vi "Locate P2.vi"(0 "Image In":T1, 11 "Error In":errorcluster, 13 "Template File Path (Locate P2 Hole)":path=path "C:/Users/serce/Desktop/Smart Vision System Testbench/P2/P2 Hole Template.png") -> (2 "Number of Matches (Locate P2 Hole)":i32, 4 "Image Dup Out":T1, 15 "Error Out":errorcluster)   [LabVIEW 2020, in "BilGör.lvlib"]
uses:
  <vilib>/vision/Image Controls.llb/IMAQ Image.ctl
  <vilib>/vision/Pattern Matching.llb/IMAQ Curve Parameters.ctl
  <vilib>/vision/Pattern Matching.llb/IMAQ Match Range Setting.ctl
  <vilib>/vision/Pattern Matching.llb/IMAQ Geometric Pattern 2 Advanced Match Options.ctl
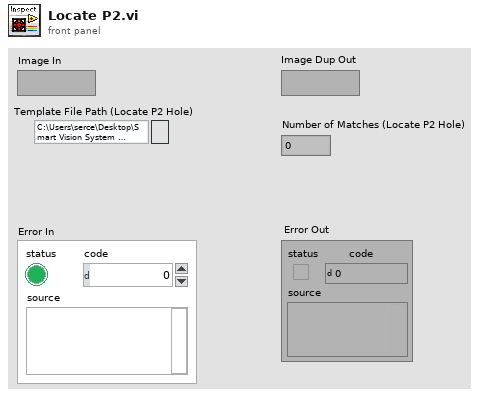
[diagram p1: front panel]
types:
  T1 = typedef "IMAQ Image.ctl" = refnum<image>
  T2 = typedef "IMAQ Curve Parameters.ctl" = cluster{"Extraction Mode":u32, "Edge Threshold":i32, "Edge Filter Size":u32, "Min Length":i32, "Row Search Step Size":i32, "Col Search Step Size":i32, "Max Endpoint Gap":i32, "Closed":bool, "Subpixel":bool}
  T3 = typedef "IMAQ Match Range Setting.ctl" = cluster{"Match Constraints":u32, "Min":dbl, "Max":dbl}
  T4 = typedef "IMAQ Geometric Pattern 2 Advanced Match Options.ctl" = u16
  T5 = cluster{"Curve Parameters":T2, "Match Mode":cluster{"Rotation":bool, "Scale":bool, "Occlusion":bool, "Reserved 1":bool, "Reserved 2":bool, "Reserved 3":bool}, "Range Settings":T3[], "Number of Matches":i32, "Minimum Match Score":sgl, "SubPixel Accuracy":bool, "Adv. Geometric Match Options 2":cluster{"Setup Data Item":T4, "Item Value":dbl}[]}
  T6 = enum16{"Reset", "Update Coordinate System", "Get Coordinate System"}
  T7 = enum16{"Horizontal Motion", "Vertical Motion", "Horizontal and Vertical Motion", "Horizontal, Vertical and Angular Motion"}
  T8 = cluster{"Origin":cluster{"X":sgl, "Y":sgl}, "Angle (deg)":sgl, "Axis Reference":u32}
  T9 = cluster{"Global Rectangle":i32[], "Contours":cluster{"ID":enum32{"External", "Internal"}, "Type":u32, "Coordinates":i32[]}[]}
  T10 = typedef "IMAQ GM Match Report.ctl" = cluster{"Position":cluster{"x":sgl, "y":sgl}, "Angle":sgl, "Scale":sgl, "Score":sgl, "Bounding Box":cluster{"x":sgl, "y":sgl}[], "Contrast Reversed":bool, "Occlusion %":sgl, "Template Target Curve Score":sgl, "Target Template Curve Score":sgl, "Correlation Score":sgl}
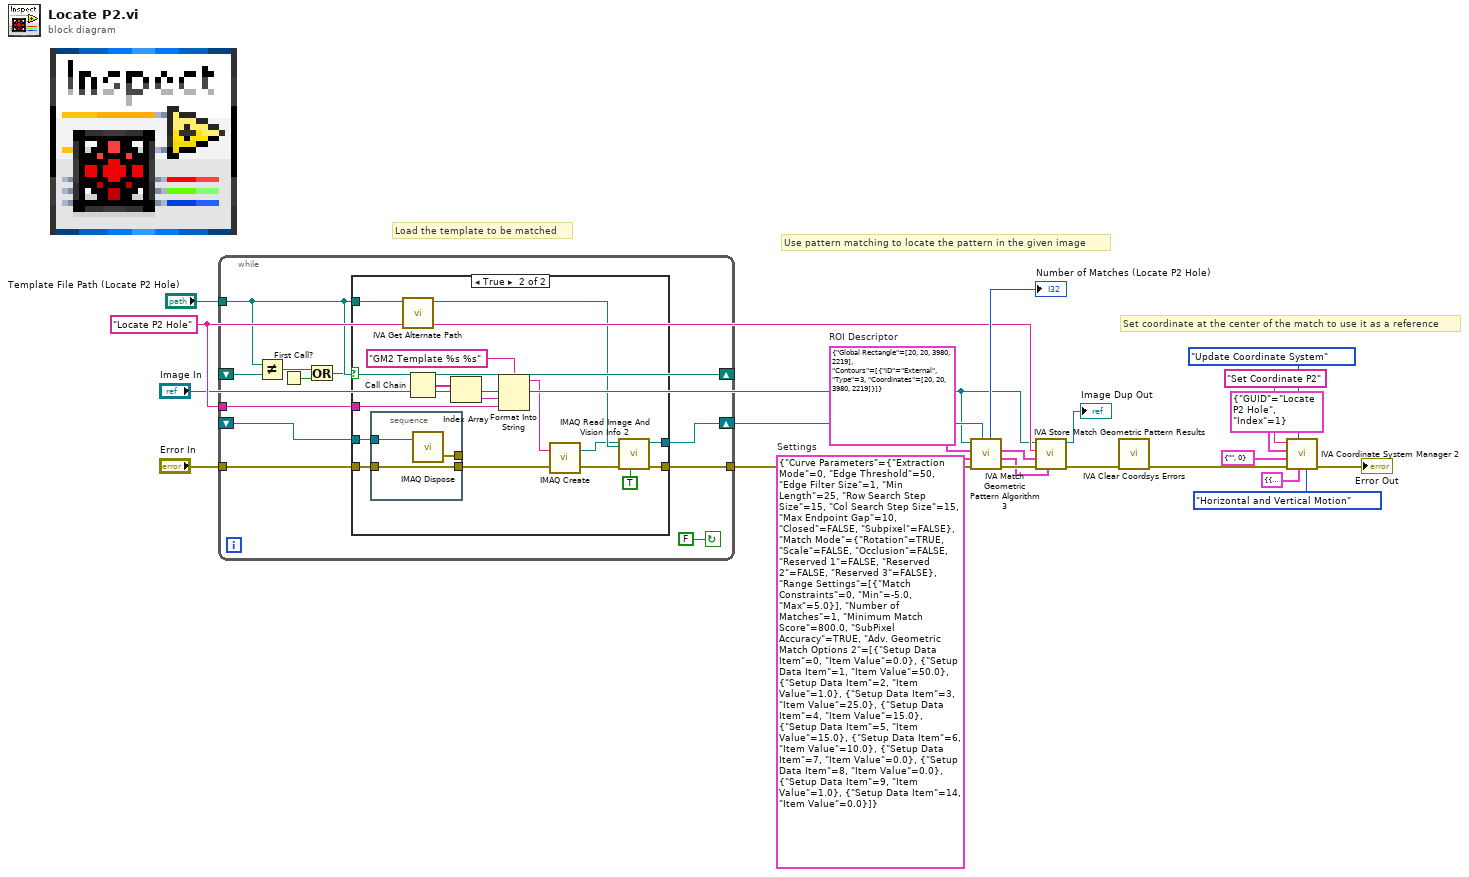
[diagram p0: block diagram]
diagram:
  w16 = T5 {"Curve Parameters"={"Extraction Mode"=0, "Edge Threshold"=50, "Edge Filter Size"=1, "Min Length"=25, "Row Search Step Size"=15, "Col Search Step Size"=15, "Max Endpoint Gap"=10, "Closed"=FALSE, "Subpixel"=FALSE}, "Match Mode"={"Rotation"=TRUE, "Scale"=FALSE, "Occlusion"=FALSE, "Reserved 1"=FALSE, "Reserved 2"=FALSE, "Reserved 3"=FALSE}, "Range Settings"=[{"Match Constraints"=0, "Min"=-5.0, "Max"=5.0}], "Number of Matches"=1, "Minimum Match Score"=800.0, "SubPixel Accuracy"=TRUE, "Adv. Geometric Match Options 2"=[{"Setup Data Item"=0, "Item Value"=0.0}, {"Setup Data Item"=1, "Item Value"=50.0}, {"Setup Data Item"=2, "Item Value"=1.0}, {"Setup Data Item"=3, "Item Value"=25.0}, {"Setup Data Item"=4, "Item Value"=15.0}, {"Setup Data Item"=5, "Item Value"=15.0}, {"Setup Data Item"=6, "Item Value"=10.0}, {"Setup Data Item"=7, "Item Value"=0.0}, {"Setup Data Item"=8, "Item Value"=0.0}, {"Setup Data Item"=9, "Item Value"=1.0}, {"Setup Data Item"=14, "Item Value"=0.0}]}  # Settings
  w15 = "Locate P2 Hole" ("Step Name")
  w21 = T9 {"Global Rectangle"=[20, 20, 3980, 2219], "Contours"=[{"ID"=enum."External", "Type"=3, "Coordinates"=[20, 20, 3980, 2219]}]}  # ROI Descriptor
  # "Set coordinate at the center of the match to use it as a reference"
  # "Use pattern matching to locate the pattern in the given image"
  # "Load the template to be matched"
  n1 = while {
    shift-right: [w33] -> w13
    shift-left: _ -> [w32]
    tunnel: [w30] -> w14
    tunnel: "Error In" -> [w29]
    tunnel: "Template File Path (Locate P2 Hole)" -> [w26]
    tunnel: w15 -> [w28]
    shift-right: [w26] -> _
    shift-left: _ -> [w27]
    stop <- FALSE continue-if-true
    n2 = Not Equal?(x=w26, y=w27) -> (x != y?=w24:bool)
    n3 = First Call?() -> (First Call?: T/F=w25:bool)
    n4 = Or(x=w24, y=w25) -> (x .or. y?=w23:bool)
    n5 = case shown="True" w23 {
      tunnel: [w35 w37] -> w33
      tunnel: w32 -> [w35 w44]
      tunnel: [w34 w39] -> w30
      tunnel: w29 -> [w34 w45]
      tunnel: w28 -> [_ w46]
      tunnel: w26 -> [_ w43]
      frame False {
      }
      frame True {
        n6 = stacked-sequence {
          tunnel: w45 -> [w53]
          tunnel: w44 -> [w52]
          tunnel: [w53] -> w42
          tunnel: [w51] -> _
          frame #0 {
            n7 = call "IMAQ Dispose"("Image"=w52) -> ("error out"=w51:errorcluster)  [unwired: 2 in, 3 out]
          }
        }
        n8 = call <vilib>:"IVA Get Alternate Path.vi"("Path In"=w43) -> ("Path Out"=w38:path)  [unwired: 10 out]
        n9 = Call Chain() -> (call chain=w48:string[])
        n10 = Index Array(array=w48) -> (element=w47:string)  [unwired: 1 in]
        n11 = Format Into String(format string="GM2 Template %s %s" ("Image Name"), w47, w46) -> (resulting string=w50:string)  [unwired: 2 in, 1 out]
        n12 = call "IMAQ Create"("Image Name"=w50, "error in (no error)"=w42) -> ("New Image"=w36:T1, "error out"=w40:errorcluster)  [unwired: 2 in, 1 out]
        n13 = call "IMAQ Read Image And Vision Info 2"("Use File Path Image Type"=TRUE, "File Path"=w38, "error in (no error)"=w40, "Image"=w36) -> ("error out"=w39:errorcluster, "Image Out"=w37:T1)  [unwired: 5 in, 1 out]
      }
    }
  }
  n14 = call <vilib>:"IVA Match Geometric Pattern Algorithm 3.vi"("Template"=w13, "error in (no error)"=w14, "Settings"=w16, "ROI Descriptor"=w21, "Image"="Image In") -> ("error out"=w20:errorcluster, "Calibrated Matches"=w18:T10[], "Matches"=w19:T10[], "Number of Matches"=→"Number of Matches (Locate P2 Hole)":i32)  [unwired: 3 out]
  n15 = call <vilib>:"IVA Store Match Geometric Pattern Results.vi"("Calibrated Matches"=w18, "error in (no error)"=w20, "Matches"=w19, "Step Name"=w15, "Image in"="Image In") -> ("error out"=w12:errorcluster, "Image dup"=→"Image Dup Out":T1)  [unwired: 5 out]
  n16 = call <vilib>:"IVA Clear Coordsys Errors.vi"("error in (no error)"=w12) -> ("error out"=w5:errorcluster)  [unwired: 10 in]
  n17 = call <vilib>:"IVA Coordinate System Manager 2.vi"("Mode"=T7."Horizontal and Vertical Motion", "Reference System"=T8 {"Origin"={"X"=2091.9944, "Y"=1085.0201}, "Angle (deg)"=0.0, "Axis Reference"=0}, "Function"=T6."Update Coordinate System", "error in (no error)"=w5, "Angle ID"=cluster{"GUID":string, "Index":i32} {"GUID"="", "Index"=0}, "Origin ID"=cluster{"GUID":string, "Index":i32} {"GUID"="Locate P2 Hole", "Index"=1}, "Coordinate System Name"="Set Coordinate P2") -> ("error out"=→"Error Out":errorcluster)  [unwired: 4 out]
